vi "test2-MacroWithSubMessages.vi"(8 "error in":errorcluster, 11 "TestCase in":refnum<class "testcase-CSMResponse.lvclass">) -> (0 "error out":errorcluster, 3 "TestCase out":refnum<class "testcase-CSMResponse.lvclass">)   [LabVIEW 2017, in "testcase-CSMResponse.lvclass"]
uses:
  testcase-CSMResponse.lvclass
  0c6454a9-3719-4e31-9ff6-45b39d38beb6.vi
  <vilib>/addons/_JKI Toolkits/VI Tester/TestCase.llb/TestCase.lvclass
  src/user.lib/_NEVSTOP/Communicable State Machine(CSM)/Communicable State Machine.lvlib
  C:/Program Files (x86)/National Instruments/LabVIEW 2017/vi.lib/addons/_JKI Toolkits/VI Tester/TestCase.llb/TestCase.lvclass
panel:
  out "Loopcount":i32
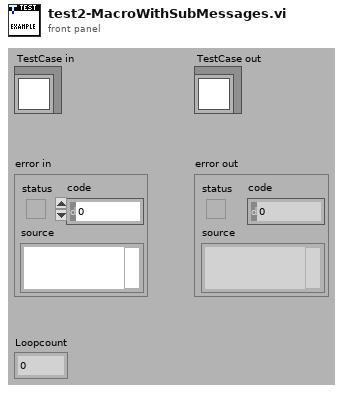
[diagram p1: front panel]
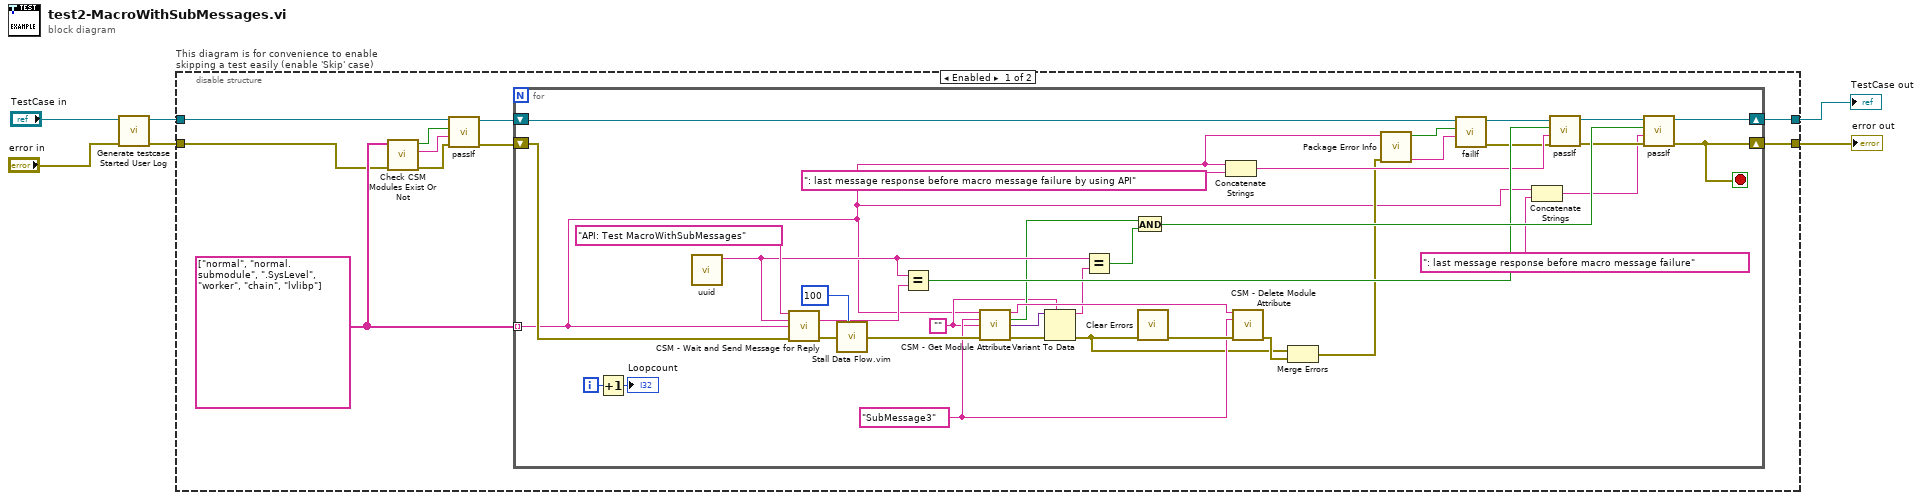
[diagram p0: block diagram]
diagram:
  n1 = call "Generate testcase Started User Log.vi"("Error In"="error in") -> ("error out"=w1:errorcluster)  [unwired: 10 in]
  n2 = disable-structure "This diagram is for convenience to enable skipping a test easily (enable 'Skip' case)" shown="Enabled" {
    disable-tunnel: "TestCase in" -> [w9 w56]
    disable-tunnel: [w15 w54] -> w2
    disable-tunnel: [w14 w55] -> w4
    disable-tunnel: w1 -> [w7 w53]
    frame Enabled {
      w10 = string[] ["normal", "normal.submodule", ".SysLevel", "worker", "chain", "lvlibp"]
      n3 = call "Check CSM Modules Exist Or Not.vi"("error in"=w7, "CSM names in"=w10) -> ("error out"=w11:errorcluster, "Debug string"=w12:string, "All Modules Exist?"=w13:bool)  [unwired: 7 in]
      n4 = call-dynamic "passIf.vi"("error in (no error)"=w11, "message (\"\")"=w12, "pass"=w13, "TestCase in"=w9) -> ("error out"=w6:errorcluster, "TestCase out"=w8:refnum<class "testcase-CSMResponse.lvclass">)  [unwired: 6 in]
      n5 = for {
        tunnel: w10 -> [w16] mode=indexing
        shift-right: [w44] -> w15
        shift-left: w8 -> [w20]
        shift-right: [w43] -> w14
        shift-left: w6 -> [w37]
        i -> [w52]
        stop <- w43 stop-if-true
        w30 = ""
        w35 = "SubMessage3" ("Attribute")
        n6 = Increment(x=w52) -> (x+1=→"Loopcount":i32)
        n7 = call "uuid.vi"() -> ("UUID"=w41:string)  [unwired: 11 in]
        n8 = call "CSM - Wait and Send Message for Reply.vi"("State"="API: Test MacroWithSubMessages", "Arguments (\"\")"=w41, "Target Module"=w16, "Error In (No Error)"=w37) -> ("Response"=w42:string, "error out"=w50:errorcluster)  [unwired: 8 in, 2 out]
        n9 = call "Stall Data Flow.vim"("value in"=w50, "milliseconds to wait"=u32 100) -> ("value out"=w36:errorcluster)  [unwired: 1 out]
        n10 = Equal?(x=w41, y=w42) -> (x = y?=w40:bool)
        n11 = call "CSM - Get Module Attribute.vi"("CSM Name"=w16, "Attribute"=w35, "Default Value (Empty Variant)"=w30, "Error In"=w36) -> ("CSM Name (Dup)"=w34:string, "Found"=w33:bool, "Value"=w31:variant, "error out"=w32:errorcluster)  [unwired: 7 in, 1 out]
        n12 = Variant To Data(error in=w32, type=w30, Variant=w31) -> (data=w29:string, error out=w27:errorcluster)
        n13 = Equal?(x=w41, y=w29) -> (x = y?=w47:bool)
        n14 = And(x=w33, y=w47) -> (x .and. y?=w46:bool)
        n15 = call <vilib>:"Clear Errors.vi"("error in (no error)"=w27) -> ("error out"=w45:errorcluster)  [unwired: 5 in, 1 out]
        n16 = Concatenate Strings(w16, ": last message response before macro message failure by using API" ("string")) -> (w25:string)
        n17 = call "CSM - Delete Module Attribute.vi"("CSM Name"=w34, "Attribute"=w35, "Error In"=w45) -> ("error out"=w28:errorcluster)  [unwired: 9 in, 3 out]
        n18 = Merge Errors(w27, w28) -> (w17:errorcluster)
        n19 = call "Package Error Info.vi"("error in"=w17, "String in"=w16) -> ("packed error info out"=w21:string, "error status"=w22:bool)  [unwired: 8 in]
        n20 = call-dynamic "failIf.vi"("message (\"\")"=w21, "fail"=w22, "TestCase in"=w20) -> ("error out"=w18:errorcluster, "TestCase out"=w19:refnum<class "testcase-CSMResponse.lvclass">)  [unwired: 7 in]
        n21 = Concatenate Strings(w16, ": last message response before macro message failure" ("string")) -> (w23:string)
        n22 = call-dynamic "passIf.vi"("error in (no error)"=w18, "message (\"\")"=w25, "pass"=w40, "TestCase in"=w19) -> ("error out"=w38:errorcluster, "TestCase out"=w39:refnum<class "testcase-CSMResponse.lvclass">)  [unwired: 6 in]
        n23 = call-dynamic "passIf.vi"("error in (no error)"=w38, "message (\"\")"=w23, "pass"=w46, "TestCase in"=w39) -> ("error out"=w43:errorcluster, "TestCase out"=w44:refnum<class "testcase-CSMResponse.lvclass">)  [unwired: 6 in]
      }
    }
    frame Disabled {
      # "skip test result while test is under development"
      n24 = call <vilib>:"skip.vi"("error in (no error)"=w53, "TestCase in"=w56) -> ("error out"=w55:errorcluster, "TestCase out"=w54:refnum<class "testcase-CSMResponse.lvclass">)  [unwired: 8 in]
    }
  }
  "error out" <- w4
  "TestCase out" <- w2
